vi "ReadKBCommand.vi"(6 "Move size (um)":dbl, 8 "handle":i32, 9 "Feedback Disable\n(Enable = TRUE)":bool, 10 "Motion #":u32, 11 "Enable\n(True)":bool) -> (0 "Enable Move\n(TRUE)":bool, 1 "Move size (mm)":dbl, 3 "Axis":enum16{"X", "Y", "Z"}(ring))   [LabVIEW 2020]
uses:
  MicroDrive.dll
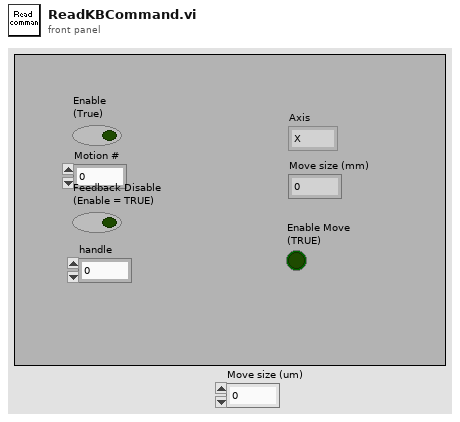
[diagram p1: front panel]
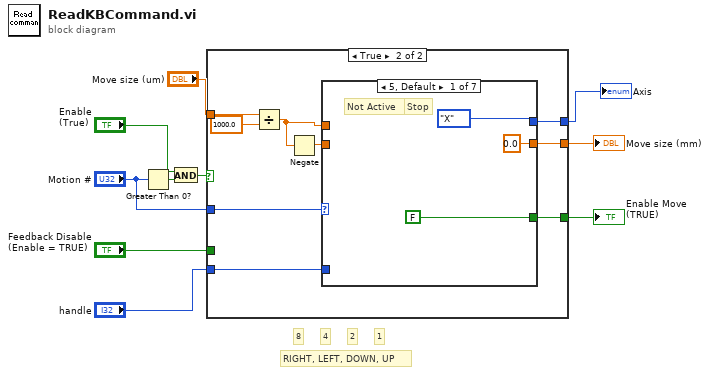
[diagram p0: block diagram]
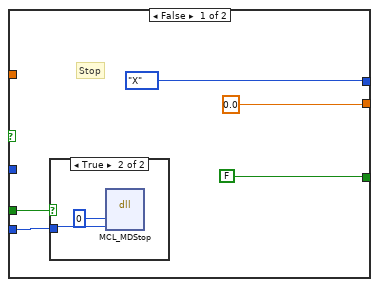
[diagram p2: hidden frame]
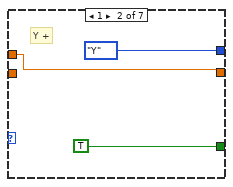
[diagram p4: hidden frame]
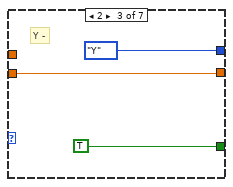
[diagram p5: hidden frame]
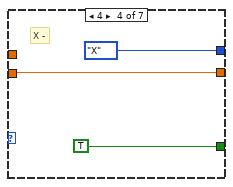
[diagram p6: hidden frame]
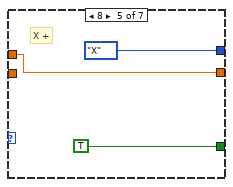
[diagram p7: hidden frame]
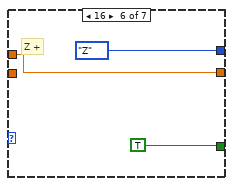
[diagram p8: hidden frame]
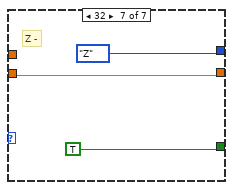
[diagram p9: hidden frame]
diagram:
  # "8"
  # "4"
  # "2"
  # "1"
  # "RIGHT, LEFT, DOWN, UP"
  n1 = Greater Than 0?(x="Motion #") -> (x > 0?=w10:bool)
  n2 = And(x="Enable\n(True)", y=w10) -> (x .and. y?=w9:bool)
  n3 = case shown="True" w9 {
    tunnel: [FALSE w26] -> w2
    tunnel: [enum16{"X", "Y", "Z"}."X" ("Axis 2") w25] -> w4
    tunnel: "handle" -> [w13 w24]
    tunnel: "Motion #" -> [_ w23]
    tunnel: [0.0 ("Move size (mm)") w22] -> w3
    tunnel: "Feedback Disable\n(Enable = TRUE)" -> [w11 _]
    tunnel: "Move size (um)" -> [_ w21]
    frame False {
      # "Stop"
      n4 = case shown="True" w11 {
        tunnel: w13 -> [_ w16]
        frame False {
        }
        frame True {
          n5 = dll-call lib="C:/Users/WalsworthGroup/Documents/Mad City Labs/MicroDrive/Labview Examples/MicroDrive.dll" fn="MCL_MDStop"("status"=u16 0, "handle"=w16) -> ()  [unwired: 4 in, 4 out]
        }
      }
    }
    frame True {
      n6 = Divide(x=w21, y=1000.0) -> (x/y=w18:dbl)
      n7 = Negate(x=w18) -> (-x=w19:dbl)
      n8 = case shown="5, Default" w23 {
        tunnel: w24 -> [_ _ _ _ _ _ _]
        tunnel: [FALSE TRUE TRUE TRUE TRUE TRUE TRUE] -> w26
        tunnel: [enum16{"X", "Y", "Z"}."X" ("Axis 2") enum16{"X", "Y"}."Y" ("Axis 2") enum16{"X", "Y"}."Y" ("Axis 2") enum16{"X", "Y"}."X" ("Axis 2") enum16{"X", "Y"}."X" ("Axis 2") enum16{"X", "Y", "Z"}."Z" ("Axis 2") enum16{"X", "Y", "Z"}."Z" ("Axis 2")] -> w25
        tunnel: [0.0 ("Move size (mm)") w30 w33 w36 w39 w42 w45] -> w22
        tunnel: w19 -> [_ _ w33 w36 _ _ w45]
        tunnel: w18 -> [_ w30 _ _ w39 w42 _]
        frame 5, Default {
          # "Stop"
          # "Not Active"
        }
        frame 1 {
          # "Y +"
        }
        frame 2 {
          # "Y -"
        }
        frame 4 {
          # "X -"
        }
        frame 8 {
          # "X +"
        }
        frame 16 {
          # "Z +"
        }
        frame 32 {
          # "Z -"
        }
      }
    }
  }
  "Axis" <- w4
  "Move size (mm)" <- w3
  "Enable Move\n(TRUE)" <- w2
